vi "HTTP_FritzBox_WebServer_DP.vi"() -> ()   [LabVIEW 2020]
doc: "HTTP SOAP Action access for a FritzBox Device (AVM Company)."
uses:
  <vilib>/Utility/error.llb/whitespace.ctl
  <vilib>/httpClient/POSTBuffer.vi
  <vilib>/httpClient/LabVIEWHTTPClient.lvlib
panel:
  in  "Stop":bool
  out "WfmChart":T1(graph)
  out "Body_GetAddInf":T2 {"u:GetAddonInfosResponse"."NewX_AVM_DE_TotalBytesReceived64" format="%_3p"; "u:GetAddonInfosResponse"."NewX_AVM_DE_TotalBytesSent64" format="%_3p"; "u:GetAddonInfosResponse"."NewTotalBytesReceived" format="%_3p"; "u:GetAddonInfosResponse"."NewTotalBytesSent" format="%_3p"; "u:GetAddonInfosResponse"."NewByteReceiveRate" format="%_3p"; "u:GetAddonInfosResponse"."NewByteSendRate" format="%_3p"}
  in  "SOAPIndex":i8
  out "Body_GetInfRes":T3 {"u:GetInfoResponse"."NewDownstreamMaxRate" format="%.3p"; "u:GetInfoResponse"."NewUpstreamMaxRate" format="%.3p"; "u:GetInfoResponse"."NewDownstreamCurrRate" format="%.3p"; "u:GetInfoResponse"."NewUpstreamCurrRate" format="%.3p"}
  out "Body_GetStaTot":T4 {"u:GetStatisticsTotalResponse"."NewTransmitBlocks" format="%.3p"; "u:GetStatisticsTotalResponse"."NewReceiveBlocks" format="%.3p"}
  out "Body_GetExtIP":T5
  out "Body_GetStaInf":T6 {"u:GetStatusInfoResponse"."NewUptime" format="%.3p"}
  out "Body_GetComLink":T7 {"u:GetCommonLinkPropertiesResponse"."NewLayer1DownstreamMaxBitRate" format="%.3p"; "u:GetCommonLinkPropertiesResponse"."NewLayer1UpstreamMaxBitRate" format="%.3p"}
  out "BodiesConcat":string
  in  "SOAP Actions":T8(array[cluster])=[{"SOAP_Header_Value"={"URL_Ext"="/igdupnp/control/WANCommonIFC1", "Value"="urn:schemas-upnp-org:service:WANCommonInterfaceConfig:1", "#"="GetAddonInfos"}}, {"SOAP_Header_Value"={"URL_Ext"="/igdupnp/control/WANCommonIFC1", "Value"="urn:schemas-upnp-org:service:WANCommonInterfaceConfig:1", "#"="GetCommonLinkProperties"}}, {"SOAP_Header_Value"={"URL_Ext"="/igdupnp/control/WANIPConn1", "Value"="urn:schemas-upnp-org:service:WANIPConnection:1", "#"="GetStatusInfo"}}, {"SOAP_Header_Value"={"URL_Ext"="/igdupnp/control/WANIPConn1", "Value"="urn:schemas-upnp-org:service:WANIPConnection:1", "#"="GetExternalIPAddress"}}, {"SOAP_Header_Value"={"URL_Ext"="/upnp/control/WanDSLIfConfig1", "Value"="urn:dslforum-org:service:WANDSLInterfaceConfig:1", "#"="GetStatisticsTotal"}}, {"SOAP_Header_Value"={"URL_Ext"="/upnp/control/WanDSLIfConfig1", "Value"="urn:dslforum-org:service:WANDSLInterfaceConfig:1", "#"="GetInfo"}}, {"SOAP_Header_Value"={"URL_Ext"="/upnp/control/wlanconfig3", "Value"="urn:dslforum-org:service:WLANConfiguration:3", "#"="GetInfo"}}, {"SOAP_Header_Value"={"URL_Ext"="/upnp/control/WanDSLIfConfig1", "Value"="urn:dslforum-org:service:WANDSLInterfaceConfig:1", "#"="X_AVM-DE_GetDSLInfo"}}, {"SOAP_Header_Value"={"URL_Ext"="/upnp/control/DeviceInfo ", "Value"="urn:dslforum-org:service:DeviceInfo:1", "#"="GetInfo"}}, {"SOAP_Header_Value"={"URL_Ext"="/upnp/control/time", "Value"="urn:dslforum-org:service:Time:1", "#"="GetInfo"}}, {"SOAP_Header_Value"={"URL_Ext"="/upnp/control/DeviceConfig", "Value"="urn:dslforum-org:service:DeviceConfig:1", "#"="GetPersistentData"}}] caption="URL SOAP Actions"
  out "ErrorOut":errorcluster
  out "BufferLength":i32=367
  out "Bodies":string[](array[string])
  out "Headers":string[](array[string])
  in  "Buffer":string="<?xml version=\"1.0\" encoding=\"utf-8\"?>\n<s:Envelope xmlns:s=\"http://schemas.xmlsoap.org/soap/envelope/\" s:encodingStyle=\"http://schemas.xmlsoap.org/soap/encoding/\">\n\t<s:Body>\n\t\t<u:GetCommonLinkPropertiesResponse xmlns:u=\"urn:schemas-upnp-org:service:WANCommonInterfaceConfig:1\">\n\t\t\t<XXXType>XXX</XXXType>\n\t\t</u:GetCommonLinkPropertiesResponse>\n\t</s:Body>\n</s:Envelope>"
  in  "FritzBox_URL":string(combo)="192.168.178.1:49000"
  # "Read FritzBox SOAP Action Web Service"
  # "ControlURL"
  # "ServiceType"
  # "Action"
  # "0"
  # "1"
  # "2"
  # "3"
  # "4"
  # "5"
  # "6"
  # "7"
  # "8"
  # "9"
  # "10"
  # "https://wiki.fhem.de/wiki/FRITZBOX#TR-064"
  # "<?xml version=\"1.0\" encoding=\"utf-8\"?>\n<s:Envelope xmlns:s=\"http://schemas.xmlsoap.org/soap/envelope/\" s:encodingStyle=\"http://schemas.xmlsoap.org/soap/encoding/\">\n\t<s:Body>\n\t\t<u:GetCommonLinkPropertiesResponse xmlns:u=\"urn:schemas-upnp-org:service:WANCommonInterfaceConfig:1\">\n\t\t\t<XXXType>XXX</XXXType>\n\t\t</u:GetCommonLinkPropertiesResponse>\n\t</s:Body>\n</s:Envelope>"
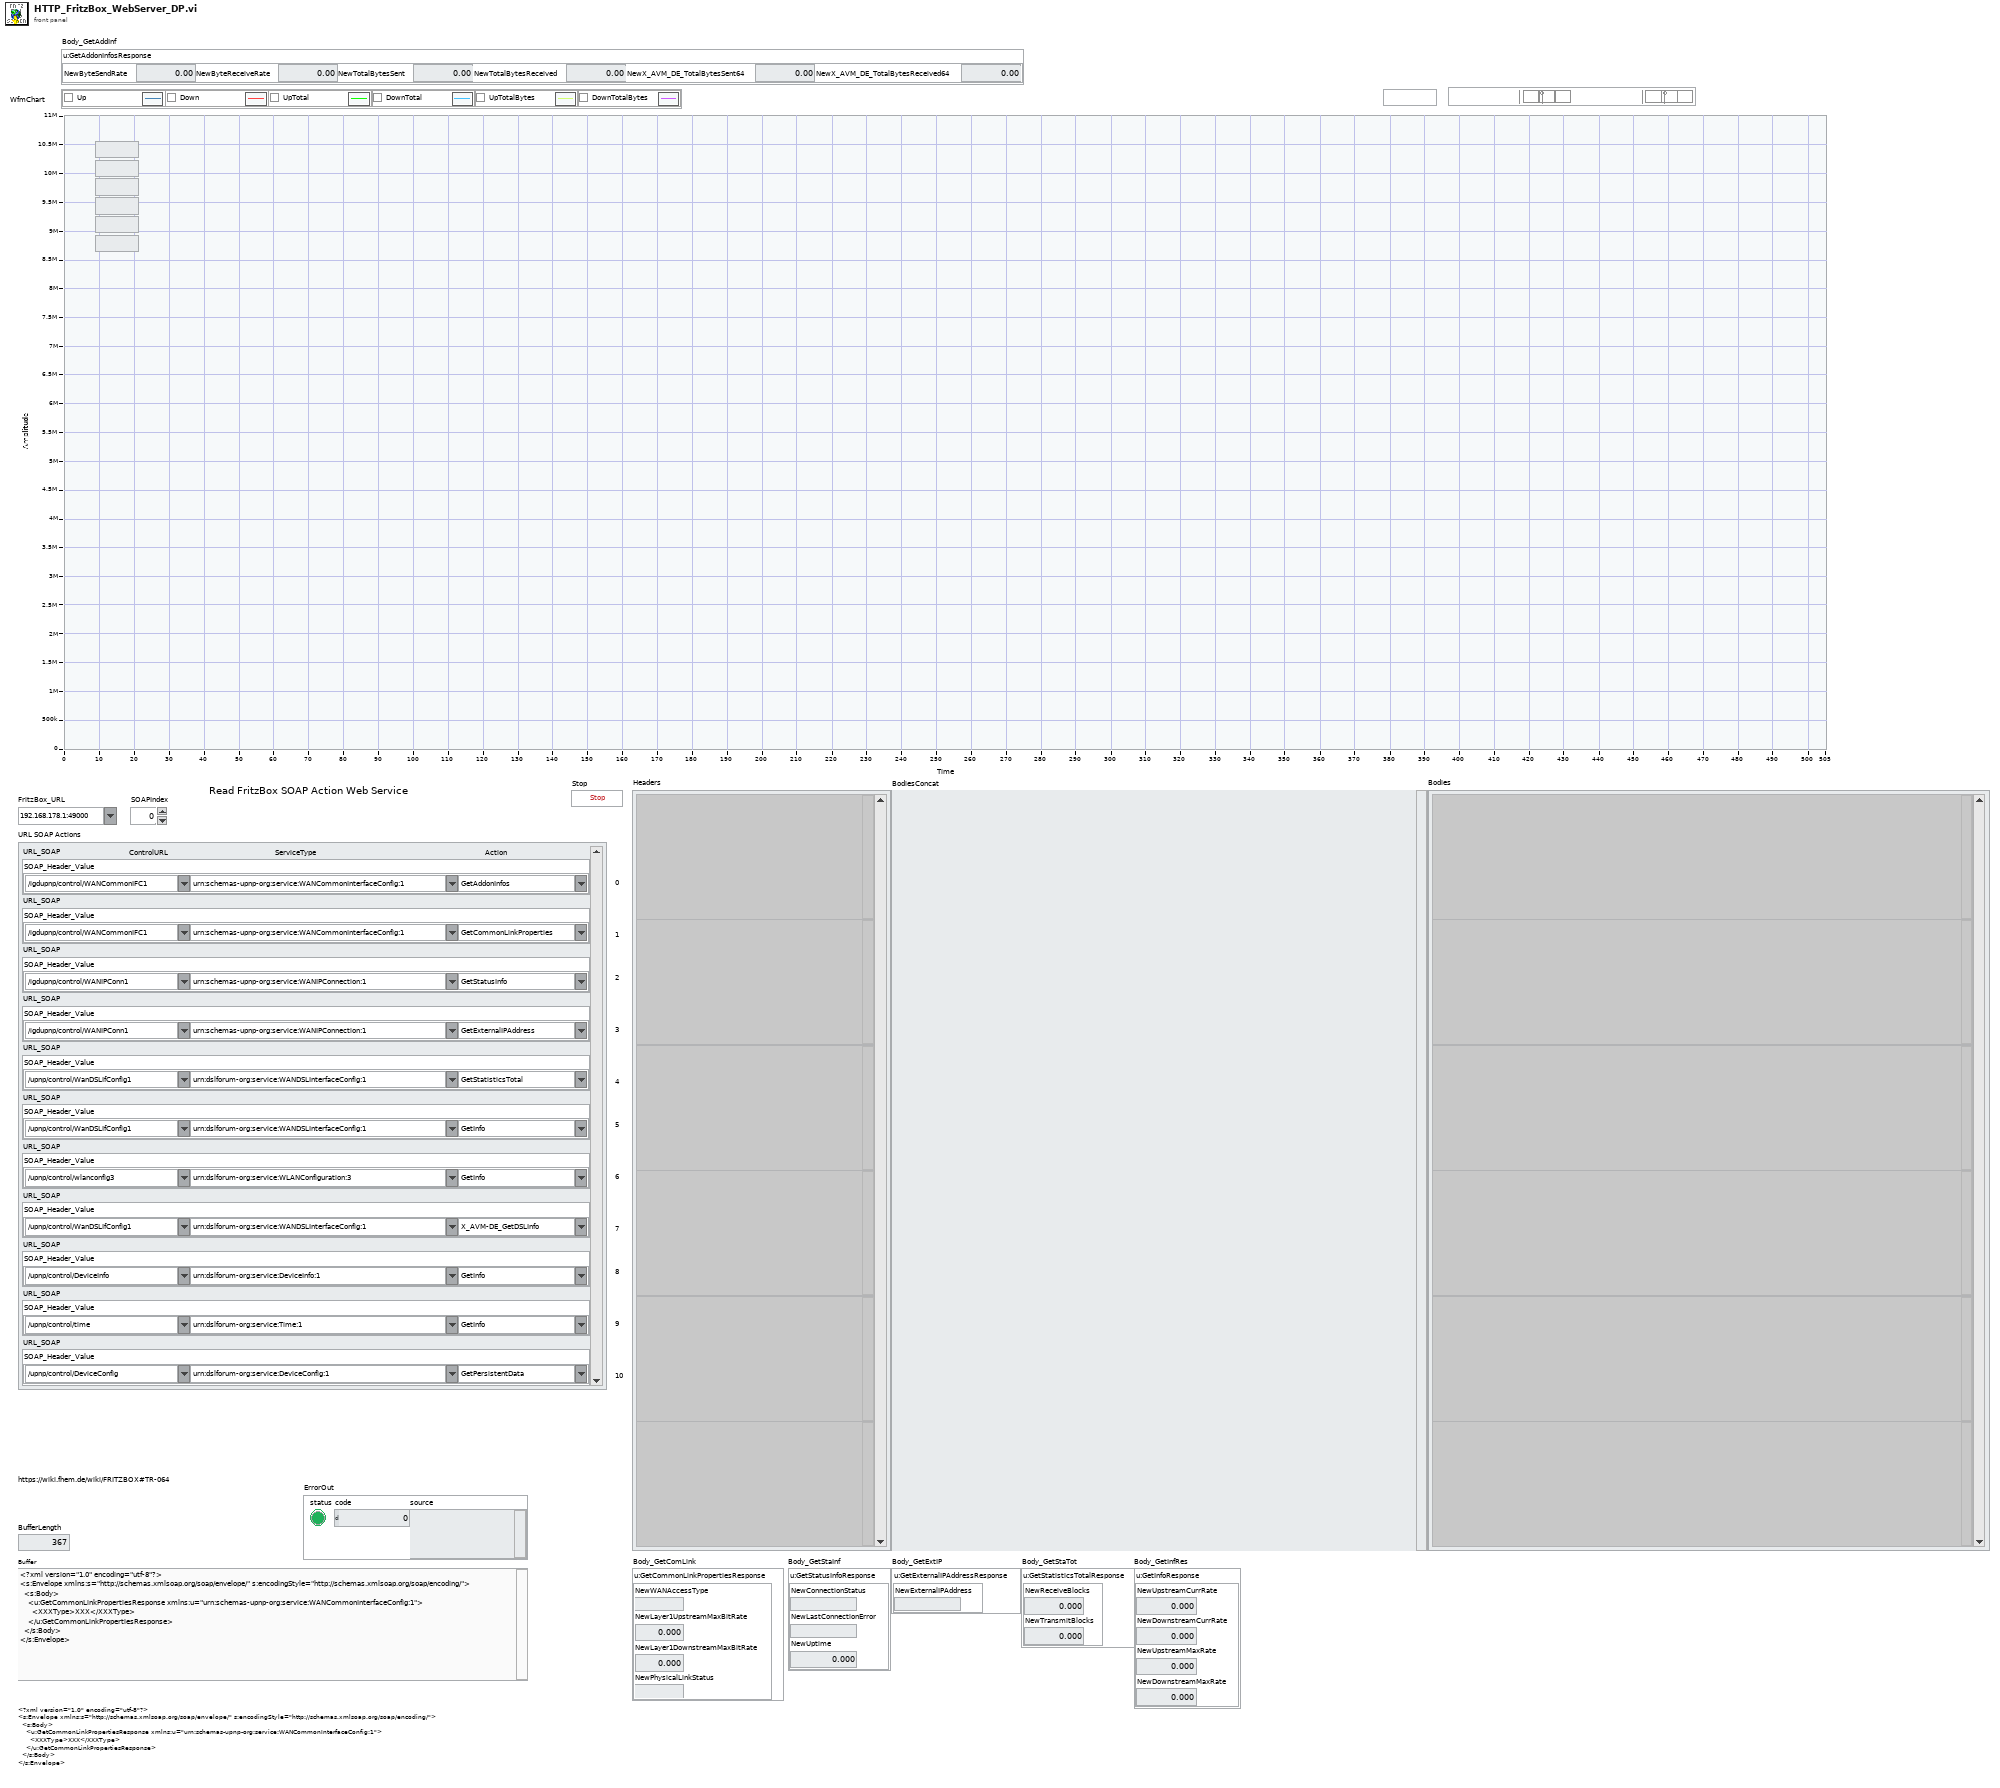
[diagram p1: front panel]
types:
  T1 = cluster{"NewByteSendRate":u32, "NewByteReceiveRate":u32, "NewTotalBytesSent":u32, "NewTotalBytesReceived":u32, "NewX_AVM_DE_TotalBytesSent64":u32, "NewX_AVM_DE_TotalBytesReceived64":u32}
  T2 = cluster{"u:GetAddonInfosResponse":cluster{"NewByteSendRate":u32, "NewByteReceiveRate":u32, "NewTotalBytesSent":u32, "NewTotalBytesReceived":u32, "NewX_AVM_DE_TotalBytesSent64":u32, "NewX_AVM_DE_TotalBytesReceived64":u32}}
  T3 = cluster{"u:GetInfoResponse":cluster{"NewUpstreamCurrRate":u32, "NewDownstreamCurrRate":u32, "NewUpstreamMaxRate":u32, "NewDownstreamMaxRate":u32}}
  T4 = cluster{"u:GetStatisticsTotalResponse":cluster{"NewReceiveBlocks":u32, "NewTransmitBlocks":u32}}
  T5 = cluster{"u:GetExternalIPAddressResponse":cluster{"NewExternalIPAddress":string}}
  T6 = cluster{"u:GetStatusInfoResponse":cluster{"NewConnectionStatus":string, "NewLastConnectionError":string, "NewUptime":u32}}
  T7 = cluster{"u:GetCommonLinkPropertiesResponse":cluster{"NewWANAccessType":string, "NewLayer1UpstreamMaxBitRate":u32, "NewLayer1DownstreamMaxBitRate":u32, "NewPhysicalLinkStatus":string}}
  T8 = cluster{"SOAP_Header_Value":cluster{"URL_Ext":string, "Value":string, "#":string}}[]
  T9 = cluster{"SOAP_Header_Value":cluster{"URL_Ext":string, "Value":string, "#":string}}
  T10 = typedef "LabVIEWHTTPClient.lvlib/ClientHandle.ctl" = refnum<k1>
  T11 = typedef "whitespace.ctl" = u16
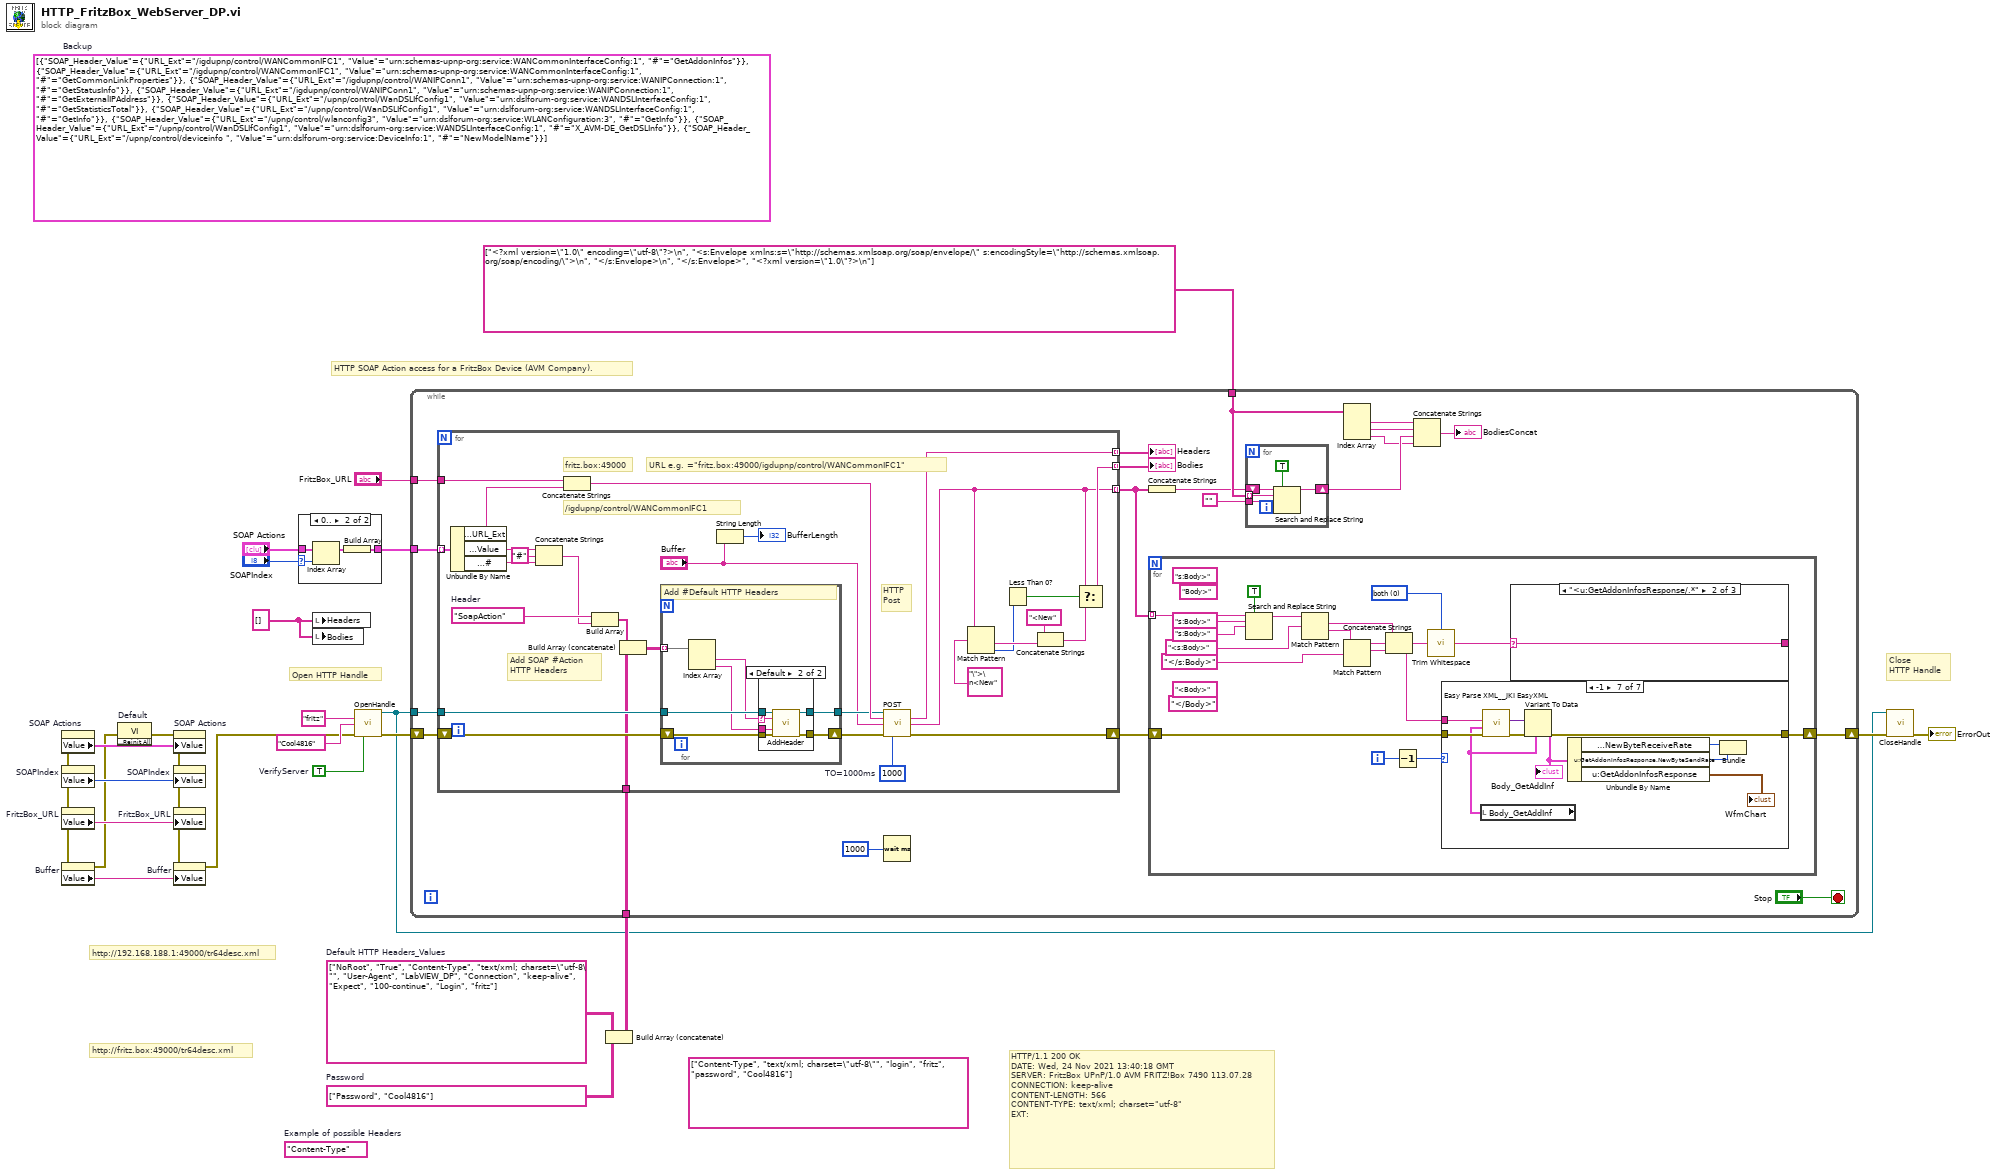
[diagram p0: block diagram]
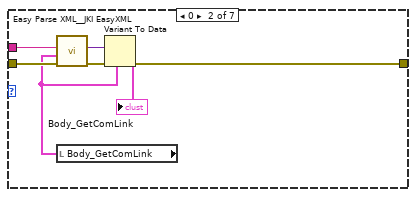
[diagram p7: hidden frame]
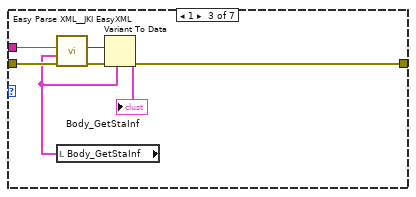
[diagram p8: hidden frame]
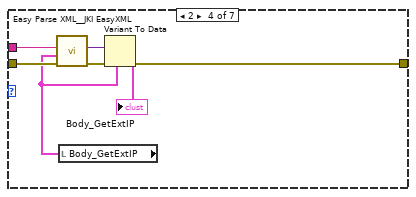
[diagram p9: hidden frame]
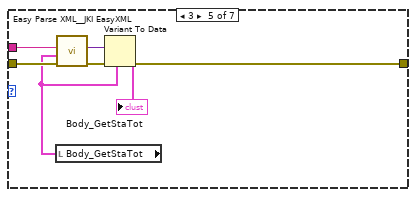
[diagram p10: hidden frame]
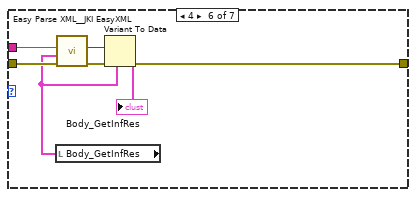
[diagram p11: hidden frame]
diagram:
  (unwired) T8 [{"SOAP_Header_Value"={"URL_Ext"="/igdupnp/control/WANCommonIFC1", "Value"="urn:schemas-upnp-org:service:WANCommonInterfaceConfig:1", "#"="GetAddonInfos"}}, {"SOAP_Header_Value"={"URL_Ext"="/igdupnp/control/WANCommonIFC1", "Value"="urn:schemas-upnp-org:service:WANCommonInterfaceConfig:1", "#"="GetCommonLinkProperties"}}, {"SOAP_Header_Value"={"URL_Ext"="/igdupnp/control/WANIPConn1", "Value"="urn:schemas-upnp-org:service:WANIPConnection:1", "#"="GetStatusInfo"}}, {"SOAP_Header_Value"={"URL_Ext"="/igdupnp/control/WANIPConn1", "Value"="urn:schemas-upnp-org:service:WANIPConnection:1", "#"="GetExternalIPAddress"}}, {"SOAP_Header_Value"={"URL_Ext"="/upnp/control/WanDSLIfConfig1", "Value"="urn:dslforum-org:service:WANDSLInterfaceConfig:1", "#"="GetStatisticsTotal"}}, {"SOAP_Header_Value"={"URL_Ext"="/upnp/control/WanDSLIfConfig1", "Value"="urn:dslforum-org:service:WANDSLInterfaceConfig:1", "#"="GetInfo"}}, {"SOAP_Header_Value"={"URL_Ext"="/upnp/control/wlanconfig3", "Value"="urn:dslforum-org:service:WLANConfiguration:3", "#"="GetInfo"}}, {"SOAP_Header_Value"={"URL_Ext"="/upnp/control/WanDSLIfConfig1", "Value"="urn:dslforum-org:service:WANDSLInterfaceConfig:1", "#"="X_AVM-DE_GetDSLInfo"}}, {"SOAP_Header_Value"={"URL_Ext"="/upnp/control/deviceinfo ", "Value"="urn:dslforum-org:service:DeviceInfo:1", "#"="NewModelName"}}]  # Backup
  w18 = string[] [] ("Headers")
  (unwired) string[][] [["Content-Type", "text/xml; charset=\"utf-8\""], ["login", "fritz"], ["password", "Cool4816"]]
  w24 = string[][] [["Password", "Cool4816"]]  # Password
  (unwired) "Content-Type"  # Example of possible Headers
  w23 = string[][] [["NoRoot", "True"], ["Content-Type", "text/xml; charset=\"utf-8\""], ["User-Agent", "LabVIEW_DP"], ["Connection", "keep-alive"], ["Expect", "100-continue"], ["Login", "fritz"]]  # Default HTTP Headers_Values
  w29 = TRUE  # VerifyServer
  # "Close \nHTTP Handle"
  # "HTTP/1.1 200 OK\nDATE: Wed, 24 Nov 2021 13:40:18 GMT\nSERVER: FritzBox UPnP/1.0 AVM FRITZ!Box 7490 113.07.28\nCONNECTION: keep-alive\nCONTENT-LENGTH: 566\nCONTENT-TYPE: text/xml; charset=\"utf-8\"\nEXT:"
  # "http://fritz.box:49000/tr64desc.xml"
  # "HTTP SOAP Action access for a FritzBox Device (AVM Company)."
  # "Open HTTP Handle"
  # "http://192.168.188.1:49000/tr64desc.xml"
  n1 = property on="SOAP Actions" class="Arr (strict)"() -> (error out=w14:errorcluster, "Value"=w15:T8)  [unwired: 2 in, 1 out]
  n2 = property on="SOAPIndex" class="DigNum (strict)"(error in=w14) -> (error out=w12:errorcluster, "Value"=w16:i8)  [unwired: 1 in, 1 out]
  n3 = property on="FritzBox_URL" class="CmbBox"(error in=w12) -> (error out=w4:errorcluster, "Value"=w10:string)  [unwired: 1 in, 1 out]
  n4 = property on="Buffer" class="Str"(error in=w4) -> (error out=w3:errorcluster, "Value"=w5:string)  [unwired: 1 in, 1 out]
  n5 = invoke on="Default" class="VI" method="Default Vals.Reinit All"(error in=w3) -> (error out=w17:errorcluster)  [unwired: 2 in, 2 out]
  n6 = property on="SOAP Actions" class="Arr (strict)"(error in=w17, "Value"=w15) -> (error out=w13:errorcluster)  [unwired: 1 in, 1 out]
  n7 = property on="SOAPIndex" class="DigNum (strict)"(error in=w13, "Value"=w16) -> (error out=w11:errorcluster)  [unwired: 1 in, 1 out]
  n8 = property on="FritzBox_URL" class="CmbBox"(error in=w11, "Value"=w10) -> (error out=w1:errorcluster)  [unwired: 1 in, 1 out]
  n9 = property on="Buffer" class="Str"(error in=w1, "Value"=w5) -> (error out=w2:errorcluster)  [unwired: 1 in, 1 out]
  n10 = case shown="0.." "SOAPIndex" {
    selector: "SOAPIndex" -> [_ w32]
    tunnel: "SOAP Actions" -> [w30 w34]
    tunnel: [w30 w31] -> w21
    frame ..-1, Default {
    }
    frame 0.. {
      n11 = Index Array(array=w34, index=w32) -> (element=w33:T9)
      n12 = Build Array(w33) -> (w31:T8)
    }
  }
  n13 = local write "Headers"(w18) -> ()
  n14 = local write "Bodies"(w18) -> ()
  n15 = call <vilib>:"OpenHandle.vi"("username"="fritz", "password"="Cool4816", "error in (no error)"=w2, "verify server(true)"=w29) -> ("client handle out"=w6:T10, "error out"=w28:errorcluster)  [unwired: 10 in]
  n16 = Build Array (concatenate)(w23, w24) -> (w19:string[][])
  n17 = while {
    tunnel: "FritzBox_URL" -> [w52]
    tunnel: w21 -> [w50]
    tunnel: w19 -> [w49]
    tunnel: string[] ["<?xml version=\"1.0\" encoding=\"utf-8\"?>\n", "<s:Envelope xmlns:s=\"http://schemas.xmlsoap.org/soap/envelope/\" s:encodingStyle=\"http://schemas.xmlsoap.org/soap/encoding/\">\n", "</s:Envelope>\n", "</s:Envelope>", "<?xml version=\"1.0\"?>\n"] ("search string") -> [w46]
    shift-right: [w38] -> w8
    shift-left: w28 -> [w53]
    tunnel: w6 -> [w35]
    stop <- "Stop" stop-if-true
    n18 = for {
      tunnel: [w71] -> w39 mode=indexing
      tunnel: w50 -> [w78] mode=indexing
      tunnel: w52 -> [w76]
      tunnel: [w83] -> w54 mode=indexing
      tunnel: w49 -> [w62]
      tunnel: [w65] -> w40 mode=indexing
      shift-right: [w80] -> w51
      shift-left: w53 -> [w81]
      tunnel: w35 -> [w82]
      w59 = "SoapAction"  # Header
      w64 = 1000  # TO=1000ms
      # "Add SOAP #Action \nHTTP Headers"
      # "HTTP \nPost"
      # "URL e.g. =\"fritz.box:49000/igdupnp/control/WANCommonIFC1\""
      # "fritz.box:49000"
      # "/igdupnp/control/WANCommonIFC1"
      n19 = Unbundle By Name(w78) -> ("SOAP_Header_Value.URL_Ext"=w60:string, "SOAP_Header_Value.Value"=w57:string, "SOAP_Header_Value.#"=w56:string)
      n20 = Concatenate Strings(w57, "#" ("string"), w56) -> (w58:string)
      n21 = Concatenate Strings(w76, w60) -> (w77:string)
      n22 = Build Array(w59, w58) -> (w61:string[])
      n23 = Build Array (concatenate)(w61, w62) -> (w63:string[][])
      n24 = for {
        shift-right: [w87] -> w74
        shift-left: w81 -> [w88]
        tunnel: w63 -> [w86] mode=indexing
        tunnel: w82 -> [w90]
        tunnel: [w89] -> w75
        # "Add #Default HTTP Headers"
        n25 = Index Array "Index Array"(array=w86) -> (element #1=w85:string, element #2=w84:string)  [unwired: 2 in]
        n26 = case shown="Default" w85 {
          selector: w85 -> [_ w94]
          tunnel: w90 -> [w91 w98]
          tunnel: [w91 w97] -> w89
          tunnel: w88 -> [w92 w96]
          tunnel: [w92 w95] -> w87
          tunnel: w84 -> [_ w93]
          frame "Connection" {
          }
          frame Default {
            n27 = call <vilib>:"AddHeader.vi"("client handle"=w98, "header"=w94, "value"=w93, "error in (no error)"=w96) -> ("client handle out"=w97:T10, "error out"=w95:errorcluster)  [unwired: 10 in]
          }
        }
      }
      n28 = String Length(string="Buffer") -> (length=→"BufferLength":i32)
      n29 = call-poly <vilib>:"POST.vi"("client handle"=w75, "url"=w77, "buffer"="Buffer", "error in (no error)"=w74, "timeout (10000)"=w64) -> ("headers"=w83:string, "body"=w65:string, "error out"=w80:errorcluster)  [unwired: 7 in, 1 out]
      n30 = Match Pattern(string=w65, regular expression="\">\n<New") -> (after substring=w70:string, offset past match=w69:i32)  [unwired: 1 in, 2 out]
      n31 = Less Than 0?(x=w69) -> (x < 0?=w68:bool)
      n32 = Concatenate Strings("<New" ("string"), w70) -> (w67:string)
      n33 = Select(t=w65, s=w68, f=w67) -> (s? t:f=w71:string)
    }
    "Headers" <- w54
    "Bodies" <- w39
    n34 = Wait (ms)(milliseconds to wait=u32 1000) -> ()  [unwired: 1 out]
    n35 = Concatenate Strings(w40) -> (w41:string)
    n36 = for {
      shift-right: [w121] -> w38
      shift-left: w51 -> [w120]
      tunnel: w40 -> [w117] mode=indexing
      i -> [w109]
      w104 = T11 0 items=["both", "start of string", "end of string"] ("location (both)")
      (unwired) "s:Body>" ("search string")
      (unwired) "</Body>" ("regular expression")
      (unwired) "<Body>" ("regular expression")
      (unwired) "Body>" ("search string")
      n37 = Search and Replace String(replace all?=TRUE ("replace all? (F)"), input string=w117, search string="s:Body>", replace string="s:Body>" ("search string")) -> (result string=w116:string)  [unwired: 4 in, 3 out]
      n38 = Match Pattern(string=w116, regular expression="<s:Body>") -> (match substring=w111:string, after substring=w112:string)  [unwired: 1 in, 2 out]
      n39 = Match Pattern(string=w112, regular expression="</s:Body>") -> (before substring=w106:string, match substring=w110:string)  [unwired: 1 in, 2 out]
      n40 = Concatenate Strings(w111, w106, w110) -> (w108:string)
      n41 = Decrement(x=w109) -> (x-1=w107:i32)
      n42 = call <vilib>:"Trim Whitespace.vi"("string"=w106, "location (both)"=w104) -> ("trimmed string"=w105:string)
      n43 = case shown="-1" w107 {
        tunnel: [w124 w130 w137 w144 w151 w158 w168] -> w121
        tunnel: w120 -> [w124 w128 w135 w142 w149 w156 w166]
        tunnel: w108 -> [_ w126 w133 w140 w147 w154 w165]
        frame Default {
        }
        frame 0 {
          n44 = local read "Body_GetComLink"() -> (w125:T7)
          n45 = call <vilib>:"Easy Parse XML__JKI EasyXML.vi"("error in (no error)"=w128, "LabVIEW Data (Type)"=w125, "XML String"=w126) -> ("error out"=w129:errorcluster, "LabVIEW Data"=w131:variant)  [unwired: 7 in]
          n46 = Variant To Data(error in=w129, type=w125, Variant=w131) -> (data=→"Body_GetComLink":T7, error out=w130:errorcluster)
        }
        frame 1 {
          n47 = local read "Body_GetStaInf"() -> (w132:T6)
          n48 = call <vilib>:"Easy Parse XML__JKI EasyXML.vi"("error in (no error)"=w135, "LabVIEW Data (Type)"=w132, "XML String"=w133) -> ("error out"=w136:errorcluster, "LabVIEW Data"=w138:variant)  [unwired: 7 in]
          n49 = Variant To Data(error in=w136, type=w132, Variant=w138) -> (data=→"Body_GetStaInf":T6, error out=w137:errorcluster)
        }
        frame 2 {
          n50 = local read "Body_GetExtIP"() -> (w139:T5)
          n51 = call <vilib>:"Easy Parse XML__JKI EasyXML.vi"("error in (no error)"=w142, "LabVIEW Data (Type)"=w139, "XML String"=w140) -> ("error out"=w143:errorcluster, "LabVIEW Data"=w145:variant)  [unwired: 7 in]
          n52 = Variant To Data(error in=w143, type=w139, Variant=w145) -> (data=→"Body_GetExtIP":T5, error out=w144:errorcluster)
        }
        frame 3 {
          n53 = local read "Body_GetStaTot"() -> (w146:T4)
          n54 = call <vilib>:"Easy Parse XML__JKI EasyXML.vi"("error in (no error)"=w149, "LabVIEW Data (Type)"=w146, "XML String"=w147) -> ("error out"=w150:errorcluster, "LabVIEW Data"=w152:variant)  [unwired: 7 in]
          n55 = Variant To Data(error in=w150, type=w146, Variant=w152) -> (data=→"Body_GetStaTot":T4, error out=w151:errorcluster)
        }
        frame 4 {
          n56 = local read "Body_GetInfRes"() -> (w153:T3)
          n57 = call <vilib>:"Easy Parse XML__JKI EasyXML.vi"("error in (no error)"=w156, "LabVIEW Data (Type)"=w153, "XML String"=w154) -> ("error out"=w157:errorcluster, "LabVIEW Data"=w159:variant)  [unwired: 7 in]
          n58 = Variant To Data(error in=w157, type=w153, Variant=w159) -> (data=→"Body_GetInfRes":T3, error out=w158:errorcluster)
        }
        frame -1 {
          n59 = local read "Body_GetAddInf"() -> (w164:T2)
          n60 = call <vilib>:"Easy Parse XML__JKI EasyXML.vi"("error in (no error)"=w166, "LabVIEW Data (Type)"=w164, "XML String"=w165) -> ("error out"=w167:errorcluster, "LabVIEW Data"=w169:variant)  [unwired: 7 in]
          n61 = Variant To Data(error in=w167, type=w164, Variant=w169) -> (data=w163:T2, error out=w168:errorcluster)
          "Body_GetAddInf" <- w163
          n62 = Unbundle By Name(w163) -> ("u:GetAddonInfosResponse.NewByteReceiveRate"=w162:u32, "u:GetAddonInfosResponse.NewByteSendRate"=w161:u32, "u:GetAddonInfosResponse"=→"WfmChart":T1)
          n63 = Bundle("NewByteReceiveRate"=w162, "NewByteSendRate"=w161) -> ()  [unwired: 1 in, 1 out]
        }
      }
      n64 = case shown="\"<u:GetAddonInfosResponse/.*\"" w105 {
        selector: w105 -> [_ w122 w123]
        tunnel: [_ w122 w123] -> _
        frame Default {
        }
        frame "<u:GetAddonInfosResponse/.*" {
        }
        frame "<u:GetCommonLinkPropertiesResponse".. {
        }
      }
    }
    n65 = for {
      tunnel: "" -> [w101]
      tunnel: w46 -> [w99] mode=indexing
      shift-right: [w100] -> w48
      shift-left: w41 -> [w102]
      n66 = Search and Replace String(replace all?=TRUE ("replace all? (F)"), input string=w102, search string=w99, replace string=w101) -> (result string=w100:string)  [unwired: 4 in, 3 out]
    }
    n67 = Index Array(array=w46) -> (element #1=w44:string, element #2=w43:string, element #3=w42:string)  [unwired: 3 in]
    n68 = Concatenate Strings(w44, w43, w48, w42) -> (→"BodiesConcat":string)
  }
  n69 = call <vilib>:"CloseHandle.vi"("client handle"=w6, "error in (no error)"=w8) -> ("error out"=→"ErrorOut":errorcluster)  [unwired: 13 in]
